vi "Read Output.vi"(0 "VISA resource name":refnum<visa-resource-name>, 5 "Address (0)":dbl min=0.0 max=31.0 step=1.0 format="%#.0p", 11 "error in (no error)":errorcluster) -> (4 "VISA resource name out":refnum<visa-resource-name>, 6 "Actual Voltage Level (V)":dbl format="%.4g", 8 "Actual Current Level (A)":dbl format="%.4g", 10 "Actual Power Level (W)":dbl format="%.4g", 14 "Output String":string, 15 "error out":errorcluster)   [LabVIEW 2020, in "BK Precision 911X Series.lvlib"]
doc: "Returns the actual voltage level and actual current level for a desired channel."
uses:
  BK Precision 911X Series.lvlib
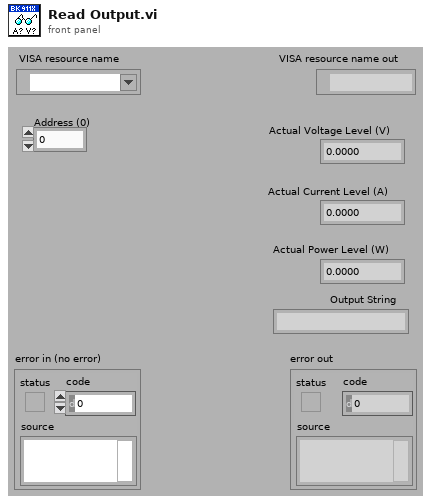
[diagram p1: front panel]
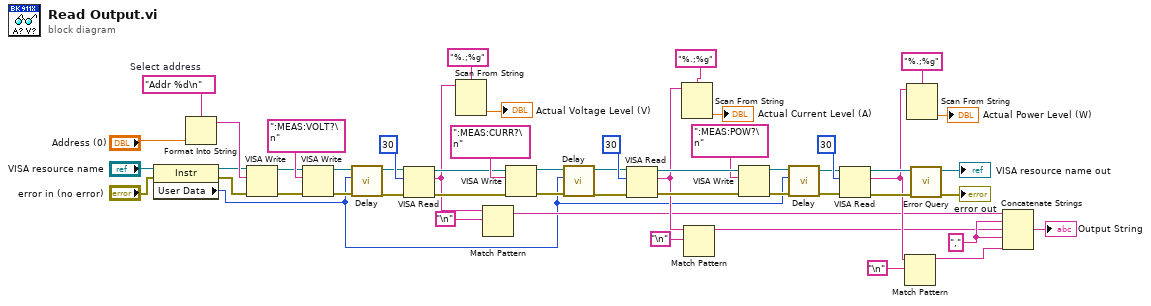
[diagram p0: block diagram]
diagram:
  w30 = ","
  w51 = "Addr %d\n"  # Select address
  n1 = property class="Instr"(reference="VISA resource name", error in="error in (no error)") -> (reference out=w15:refnum<visa-resource-name>, error out=w14:errorcluster, "User Data"=w1:u32)
  n2 = Format Into String(format string=w51, "Address (0)") -> (resulting string=w50:string)  [unwired: 2 in, 1 out]
  n3 = VISA Write(VISA resource name=w15, write buffer=w50, error in (no error)=w14) -> (VISA resource name out=w34:refnum<visa-resource-name>, error out=w33:errorcluster)  [unwired: 1 out]
  n4 = VISA Write(VISA resource name=w34, write buffer=":MEAS:VOLT?\n", error in (no error)=w33) -> (VISA resource name out=w13:refnum<visa-resource-name>, error out=w12:errorcluster)  [unwired: 1 out]
  n5 = call "Delay.vi"("error in (no error)"=w12, "Delay Time (0 ms)"=w1, "VISA resource name"=w13) -> ("error out"=w10:errorcluster, "VISA resource name out"=w11:refnum<visa-resource-name>)  [unwired: 7 in]
  n6 = VISA Read(VISA resource name=w11, byte count=30, error in (no error)=w10) -> (VISA resource name out=w44:refnum<visa-resource-name>, read buffer=w29:string, error out=w43:errorcluster)  [unwired: 1 out]
  n7 = Scan From String(format string="%.;%g", input string=w29) -> (output 1=→"Actual Voltage Level (V)":dbl)  [unwired: 3 in, 3 out]
  n8 = Match Pattern(string=w29, regular expression="\n") -> (before substring=w23:string)  [unwired: 1 in, 3 out]
  n9 = VISA Write(VISA resource name=w44, write buffer=":MEAS:CURR?\n", error in (no error)=w43) -> (VISA resource name out=w9:refnum<visa-resource-name>, error out=w8:errorcluster)  [unwired: 1 out]
  n10 = call "Delay.vi"("error in (no error)"=w8, "Delay Time (0 ms)"=w1, "VISA resource name"=w9) -> ("error out"=w6:errorcluster, "VISA resource name out"=w7:refnum<visa-resource-name>)  [unwired: 7 in]
  n11 = VISA Read(VISA resource name=w7, byte count=30, error in (no error)=w6) -> (VISA resource name out=w39:refnum<visa-resource-name>, read buffer=w24:string, error out=w38:errorcluster)  [unwired: 1 out]
  n12 = Scan From String(format string="%.;%g", input string=w24) -> (output 1=→"Actual Current Level (A)":dbl)  [unwired: 3 in, 3 out]
  n13 = Match Pattern(string=w24, regular expression="\n") -> (before substring=w22:string)  [unwired: 1 in, 3 out]
  n14 = VISA Write(VISA resource name=w39, write buffer=":MEAS:POW?\n", error in (no error)=w38) -> (VISA resource name out=w5:refnum<visa-resource-name>, error out=w4:errorcluster)  [unwired: 1 out]
  n15 = call "Delay.vi"("error in (no error)"=w4, "Delay Time (0 ms)"=w1, "VISA resource name"=w5) -> ("error out"=w3:errorcluster, "VISA resource name out"=w2:refnum<visa-resource-name>)  [unwired: 7 in]
  n16 = VISA Read(VISA resource name=w2, byte count=30, error in (no error)=w3) -> (VISA resource name out=w35:refnum<visa-resource-name>, read buffer=w25:string, error out=w36:errorcluster)  [unwired: 1 out]
  n17 = Match Pattern(string=w25, regular expression="\n") -> (before substring=w21:string)  [unwired: 1 in, 3 out]
  n18 = Scan From String(format string="%.;%g", input string=w25) -> (output 1=→"Actual Power Level (W)":dbl)  [unwired: 3 in, 3 out]
  n19 = call "Error Query.vi"("error in (no error)"=w36, "VISA resource name"=w35) -> ("error out"=→"error out":errorcluster, "VISA resource name out"=→"VISA resource name out":refnum<visa-resource-name>)  [unwired: 6 in, 2 out]
  n20 = Concatenate Strings(w23, w30, w22, w30, w21) -> (→"Output String":string)
